vi "4Pi Interference Locator NEW.vi"(7 "Calling VI Ref":refnum<vi>) -> ()   [LabVIEW 2016]
uses:
  <vilib>/vision/Image Controls.llb/IMAQ Image.ctl
  Hardware Configuration/Hardware Configuration Controls/Device Type.ctl
  Hardware Configuration/Hardware Configuration Controls/Device Function.ctl
  Device Library/Stages/Stages Controls/Stage Actions.ctl
  <vilib>/Utility/miscctls.llb/LVPointTypeDef.ctl
  4Pi Interference Locator Type Defs/4Pi IL Notifier Type.ctl
  4Pi Interference Locator Type Defs/4Pi IL Actions.ctl
  Device Manager/Common Device Queue/Common Device Controls/Common Device Actions.ctl
  Device Library/Cameras/Hamamatsu/Orca Flash/Orca Flash Controls/Orca Flash Actions.ctl
  Display Module/Display Module Custom Controls/ROI Descriptor.ctl
  Device Library/Stages/Stages Controls/Stage Status.ctl
  <vilib>/vision/NI_Vision_Development_Module.lvlib
panel:
  in  "Move to Cursor":bool
  in  "Halt Stage":bool
  in  "Scan Range (µm)":dbl
  out "Interference Scan":cluster{sgl[], sgl[]}(graph)
  in  "Clear Plot":bool=TRUE
  in  "Stage Settings":bool
  in  "Scan Cavity":bool
  in  "Velocity":dbl=0.001
  in  "Quit":bool
  in  "Interference Image":i32(ring) items=["Quad 01", "Quad 02", "Quad 03", "Quad 04"]
  in  "Cavity Position (µm)":dbl
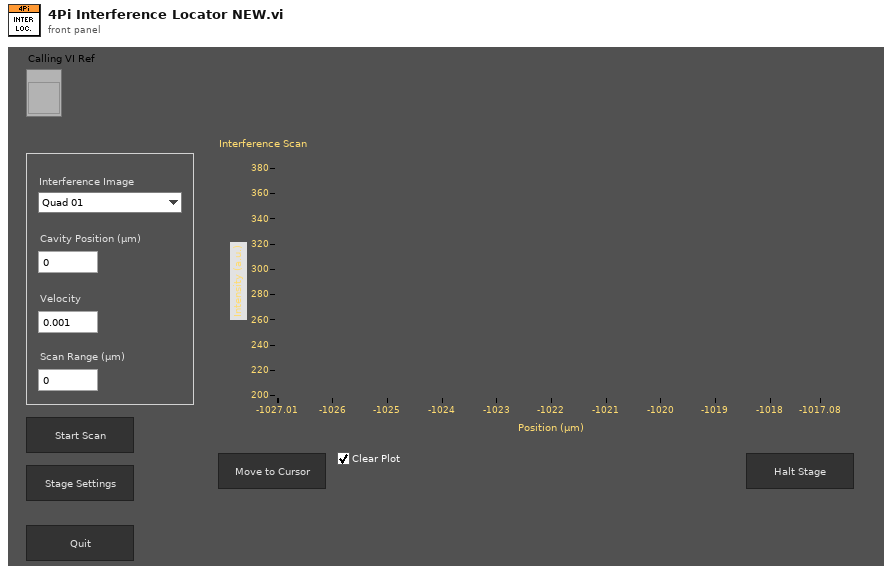
[diagram p1: front panel]
types:
  T1 = typedef "4Pi IL Actions.ctl" = enum16{"Idle", "Start Scan", "Move Stage", "Get Data", "Wait For Update", "Abort", "End Scan", "Quit"}
  T2 = typedef "4Pi IL Notifier Type.ctl" = cluster{"Actions":T1, "Image Ref":T3, "Scan Image Mask":T3}
  T3 = typedef "IMAQ Image.ctl" = refnum<image>
  T4 = enum16{"Always On", "Always Off", "Off While Running"}
  T5 = typedef "LVPointTypeDef.ctl" = cluster{"Horizontal":i16, "Vertical":i16}
  T6 = typedef "Stage Actions.ctl" = enum16{"Get Position", "MVR", "MOVE", "HALT", "ONTARGET", "ERROR", "REFERENCE", "INIT", "VELOCITY", "STATUS", "EXIT", "HOME", "ZEROPOS", "NANOPOS", "ANALOG", "QUIT"}
  T7 = typedef "Image Type" = u32
  T8 = typedef "Device Function.ctl" = enum16{"Primary", "Secondary", "Overview", "Wide Field Drift Correction", "642 nm Excitation", "560 nm Excitation", "546 nm Excitation", "488 nm Excitation", "405 nm Excitation", "Objective Drift Correction", "Objective XY", "Objective Z", "Sample XY", "Sample Coarse Z", "Sample Z", "4Pi Lower", "4Pi Upper", "Adj Cavity", "Line Scanning"}
  T9 = typedef "Device Type.ctl" = enum16{"AOTF", "Camera", "Deformable Mirror", "Laser", "Shutter", "Stage", "Waveform"}
  T10 = typedef "ROI Descriptor.ctl" = cluster{"Global Rectangle":i32[], "Contours":cluster{"Contour Type":u32, "ROI Type":u32, "Points":i32[]}[]}
  T11 = typedef "Orca Flash Actions.ctl" = enum16{"IDLE", "PREVIEW", "RECORD", "Record Settings", "SETPARAM", "GETPARAM", "SETROI", "GETROI", "PROGRESSIVE MODE", "AREA MODE", "STATUS", "QUIT"}
  T12 = typedef "Stage Status.ctl" = enum16{"Error", "Abort", "Busy", "On Target"}
  T13 = typedef "Common Device Actions.ctl" = enum16{"Open Front Panel", "Close Front Panel", "Quit", "Quit All"}
  T14 = cluster{"Contour Type":u32, "ROI Type":u32, "Points":i32[]}[]
  T15 = cluster{"Contour Type":u32, "ROI Type":u32, "Points":i32[]}
  T16 = cluster{"Mean Value":sgl, "Standard Variation":sgl, "Minimal Value":sgl, "Maximal Value":sgl, "Area (calibrated)":sgl, "Area (pixels)":u32, "%":sgl, "Calibration Valid":bool}
  T17 = typedef "LVRectTypeDef.ctl" = cluster{"Left":i16, "Top":i16, "Right":i16, "Bottom":i16}
  T18 = typedef "LVBoundsTypeDef.ctl" = cluster{"Width":u32, "Height":u32}
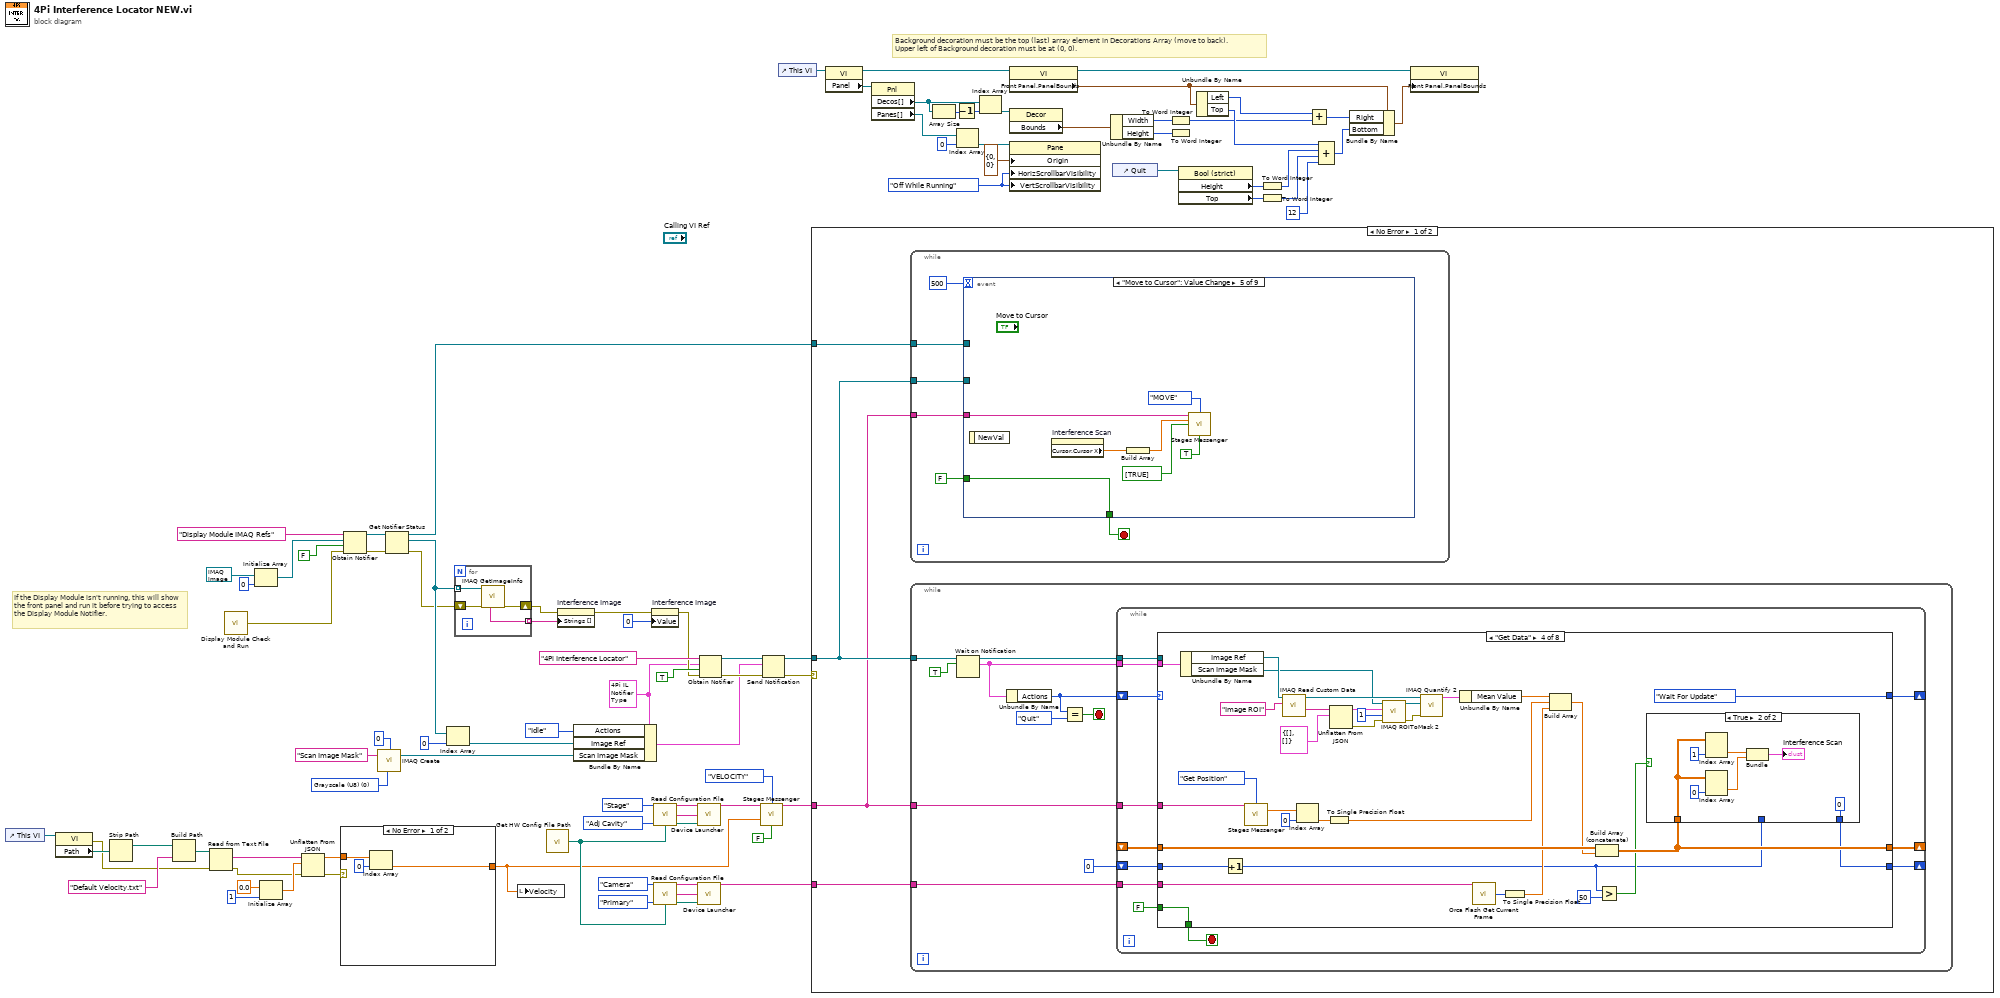
[diagram p0: block diagram]
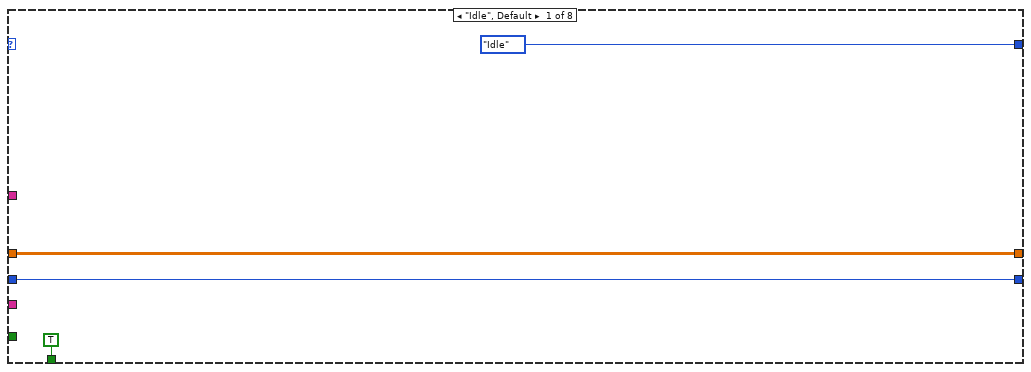
[diagram p2: hidden frame]
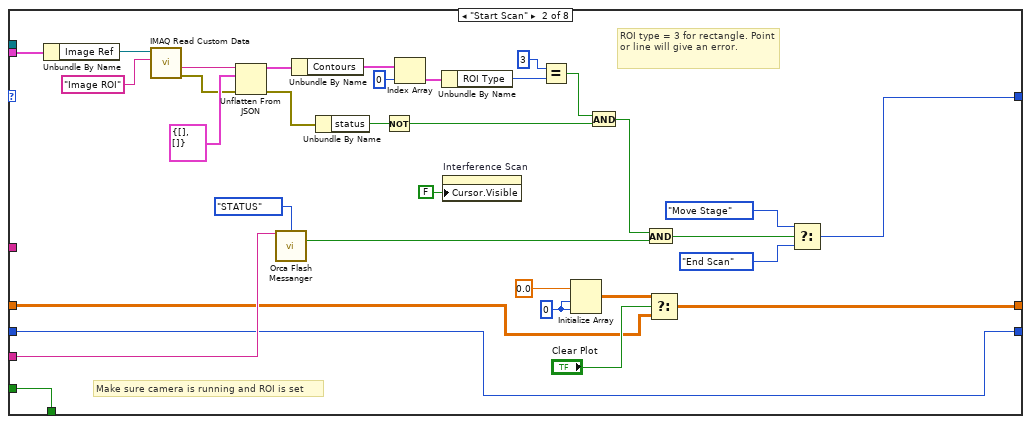
[diagram p3: hidden frame]
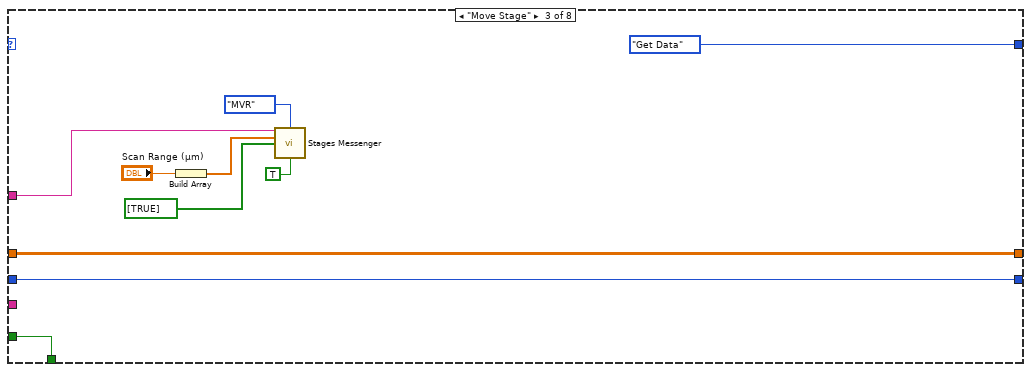
[diagram p4: hidden frame]
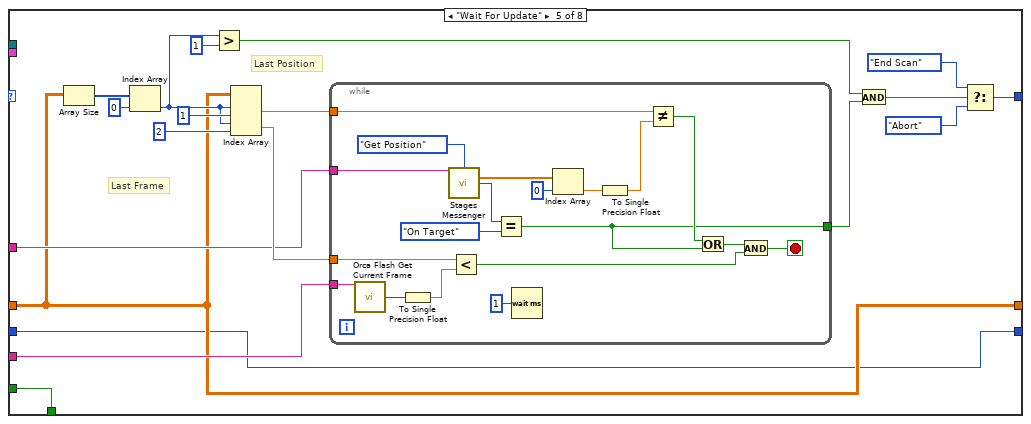
[diagram p6: hidden frame]
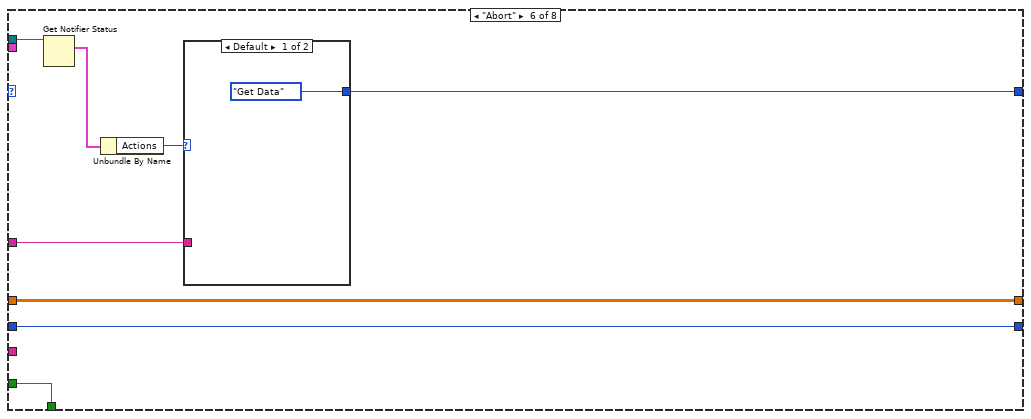
[diagram p7: hidden frame]
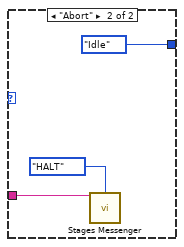
[diagram p8: hidden frame]
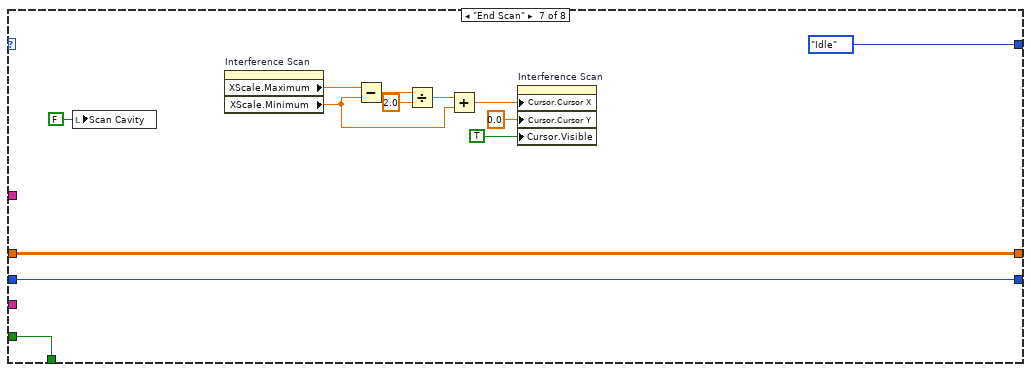
[diagram p9: hidden frame]
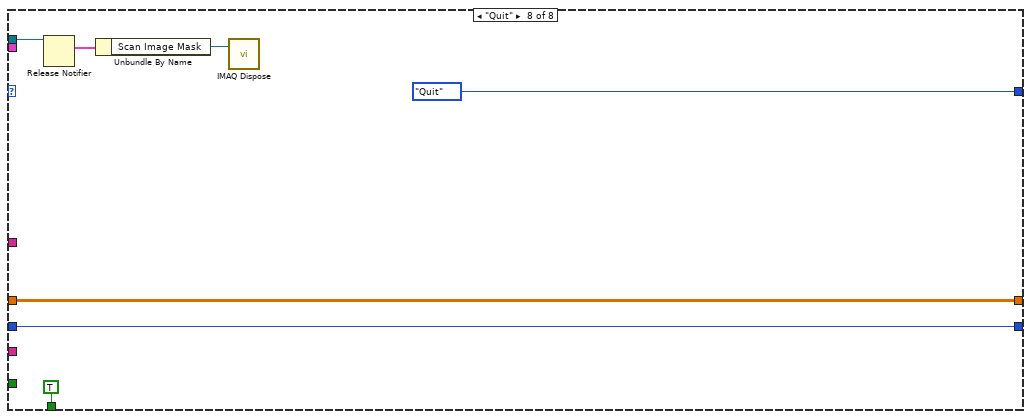
[diagram p10: hidden frame]
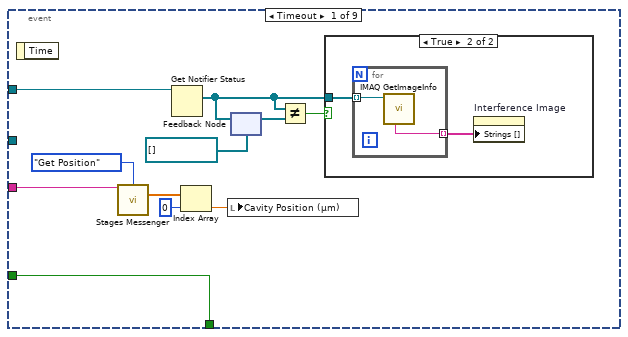
[diagram p11: hidden frame]
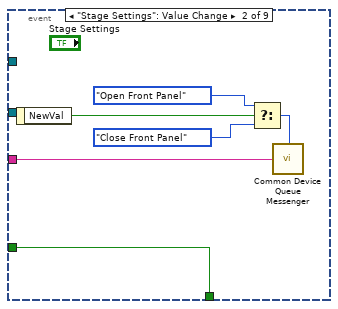
[diagram p13: hidden frame]
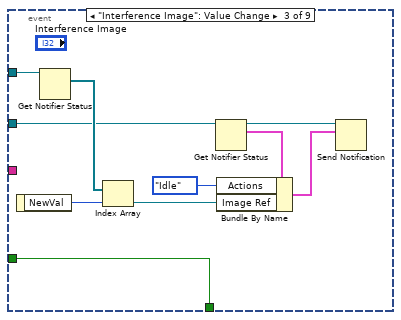
[diagram p14: hidden frame]
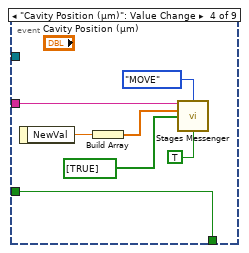
[diagram p15: hidden frame]
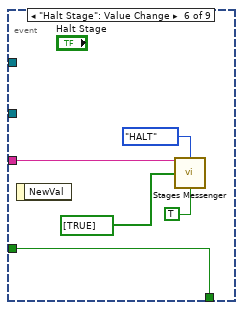
[diagram p16: hidden frame]
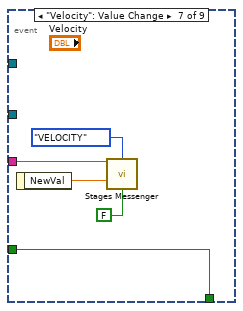
[diagram p17: hidden frame]
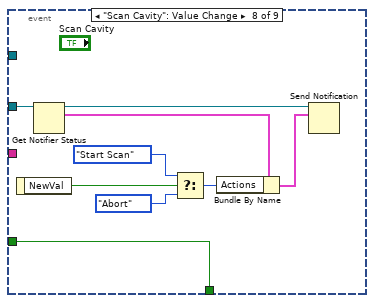
[diagram p18: hidden frame]
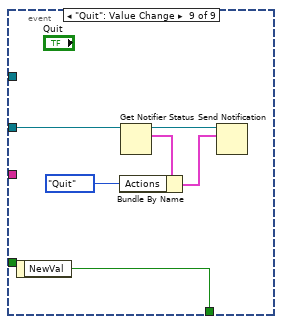
[diagram p19: hidden frame]
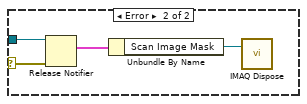
[diagram p20: hidden frame]
diagram:
  w9 = T2 {"Actions"=enum."Idle", "Image Ref"=refnum, "Scan Image Mask"=refnum} ("4Pi IL Notifier Type")
  w49 = T4."Off While Running" ("Vertical Scrollbar Visibility")
  w71 = T7 0 items=["Grayscale (U8)", "Grayscale (I16)", "Grayscale (SGL)", "Complex (CSG)", "RGB (U32)", "HSL (U32)", "RGB (U64)", "Grayscale (U16)"] ("Image Type")
  # "If the Display Module isn't running, this will show the front panel and run it before trying to access the Display Module Notifier."
  # "Background decoration must be the top (last) array element in Decorations Array (move to back).\nUpper left of Background decoration must be at (0, 0)."
  n1 = control-ref of="This VI"() -> (w37:refnum<vi>)
  n2 = property class="VI"(reference=w37) -> (error out=w28:errorcluster, "Path"=w36:path)  [unwired: 1 in, 1 out]
  n3 = Strip Path(path=w36) -> (stripped path=w29:path)  [unwired: 1 out]
  n4 = Build Path(base path=w29, name or relative path="Default Velocity.txt") -> (appended path=w31:path)
  n5 = Read from Text File(file (use dialog)=w31, error in=w28) -> (text=w30:string, error out=w27:errorcluster)  [unwired: 2 in, 2 out]
  n6 = call "Display Module Check and Run.vi"() -> ("Error"=w23:errorcluster)  [unwired: 15 in]
  n7 = Initialize Array(T3 refnum ("New Image"), 0 ("dimension size")) -> (w86:T3[])
  n8 = Initialize Array(0.0 ("element"), 1 ("dimension size")) -> (w32:dbl[])
  n9 = Unflatten From JSON(JSON string=w30, type and defaults=w32, error in (no error)=w27) -> (value=w25:dbl[], error out=w26:errorcluster)  [unwired: 4 in]
  n10 = case shown="No Error" w26 {
    tunnel: w25 -> [w92 _]
    tunnel: [w91 1.0 ("element")] -> w24
    frame No Error {
      n11 = Index Array(array=w92, index=0) -> (element=w91:dbl)
    }
    frame Error {
      n12 = One Button Dialog(message="Default cavity stage velocity not found in 4Pi Interference Locator. Please set this value") -> ()  [unwired: 1 in, 1 out]
    }
  }
  n13 = Obtain Notifier(name (unnamed)="Display Module IMAQ Refs", notification data type=w86, create if not found? (T)=FALSE, error in (no error)=w23) -> (notifier out=w85:refnum<notifier>, error out=w22:errorcluster)  [unwired: 1 out]
  n14 = call "IMAQ Create"("Border Size"=0, "Image Name"="Scan Image Mask", "Image Type"=w71) -> ("New Image"=w1:T3)  [unwired: 2 in, 1 out]
  n15 = Get Notifier Status(notifier=w85, error in (no error)=w22) -> (notifier out=w2:refnum<notifier>, current notification=w20:T3[], error out=w19:errorcluster)  [unwired: 2 out]
  n16 = Index Array(array=w20, index=0) -> (element=w7:T3)
  n17 = for {
    tunnel: w20 -> [w99] mode=indexing
    shift-right: [w97] -> w14
    shift-left: w19 -> [w98]
    tunnel: [w96] -> w18 mode=indexing
    n18 = call "IMAQ GetImageInfo"("error in (no error)"=w98, "Image"=w99) -> ("error out"=w97:errorcluster, "Image Name"=w96:string)  [unwired: 2 in, 6 out]
  }
  n19 = local write "Velocity"(w24) -> ()
  n20 = call "Get HW Config File Path.vi"() -> ("File Path"=w73:path)  [unwired: 14 in, 1 out]
  n21 = property on="Interference Image" class="Ring (strict)"(error in=w14, "Strings []"=w18) -> (error out=w21:errorcluster)  [unwired: 1 in, 1 out]
  n22 = Bundle By Name(cluster=w9, "Actions"=4Pi_IL_Actions."Idle", "Image Ref"=w7, "Scan Image Mask"=w1) -> (w6:T2)
  n23 = property on="Interference Image" class="Ring (strict)"(error in=w21, "Value"=0) -> (error out=w13:errorcluster)  [unwired: 1 in, 1 out]
  n24 = call "Read Configuration File.vi"("Device Type"=Device_Type."Stage", "Device Function"=Device_Function."Adj Cavity", "Config File Path"=w73) -> ("Unique Notifier Name"=w83:string, "Device Ports/IDs/Channels"=w81:string[], "Device Engine Path"=w82:path)  [unwired: 9 in, 1 out]
  n25 = call "Read Configuration File.vi"("Device Type"=Device_Type."Camera", "Device Function"=Device_Function."Primary", "Config File Path"=w73) -> ("Unique Notifier Name"=w74:string, "Device Ports/IDs/Channels"=w76:string[], "Device Engine Path"=w75:path)  [unwired: 9 in, 1 out]
  n26 = call "Device Launcher.vi"("Notifier Name"=w83, "Device Ports/IDs/Channels"=w81, "Device Engine Path"=w82) -> ("Notifier Name"=w67:string)  [unwired: 11 in, 1 out]
  n27 = call "Device Launcher.vi"("Notifier Name"=w74, "Device Ports/IDs/Channels"=w76, "Device Engine Path"=w75) -> ("Notifier Name"=w3:string)  [unwired: 11 in, 1 out]
  n28 = Obtain Notifier(name (unnamed)="4Pi Interference Locator", notification data type=w9, create if not found? (T)=TRUE, error in (no error)=w13) -> (notifier out=w12:refnum<notifier>, error out=w11:errorcluster)  [unwired: 1 out]
  n29 = call "Stages Messenger.vi"("Stage Notifier Name"=w67, "Actions"=Stage_Actions."VELOCITY", "Velocity"=w24, "Exit While Busy?"=FALSE) -> ("Stage Notifier Name (Dup)"=w4:string)  [unwired: 8 in, 3 out]
  n30 = Send Notification(notification=w6, notifier=w12, error in (no error)=w11) -> (notifier out=w5:refnum<notifier>, error out=w10:errorcluster)
  n31 = control-ref of="This VI"() -> (w41:refnum<vi>)
  n32 = case shown="No Error" w10 {
    selector: w10 -> [_ w361]
    tunnel: w5 -> [w103 w362]
    tunnel: w4 -> [w101 _]
    tunnel: w3 -> [w102 _]
    tunnel: w2 -> [w100 _]
    frame No Error {
      n33 = while {
        tunnel: w103 -> [w286]
        tunnel: w101 -> [w285]
        tunnel: w100 -> [w284]
        stop <- w288 stop-if-true
        n34 = event shown="[4] \"Move to Cursor\": Value Change" {
          selector: _ -> [_ _ _ _ _ _ _ _ _]
          dyn-events: _ -> [_ _ _ _ _ _ _ _ _]
          timeout: 500 -> [_ _ _ _ _ _ _ _ _]
          tunnel: w284 -> [w300 _ w319 _ _ _ _ _ _]
          tunnel: [w296 w310 w320 w327 w334 w339 w344 w348 w359] -> w288
          tunnel: FALSE -> [w296 w310 w320 w327 w334 w339 w344 w348 _]
          tunnel: w285 -> [w295 w306 _ w324 w332 w337 w341 _ _]
          tunnel: w286 -> [_ _ w316 _ _ _ _ w352 w358]
          event Timeout {
            n35 = event-data() -> ()  [unwired: 1 in, 1 out]
            n36 = call "Stages Messenger.vi"("Stage Notifier Name"=w295, "Actions"=Stage_Actions."Get Position") -> ("Positions"=w293:dbl[])  [unwired: 10 in, 3 out]
            n37 = Get Notifier Status(notifier=w300) -> (current notification=w297:T3[])  [unwired: 1 in, 4 out]
            n38 = Index Array(array=w293, index=0) -> (element=w291:dbl)
            n39 = local write "Cavity Position (µm)"(w291) -> ()
            n40 = feedback-in #1(w297) -> ()
            n41 = feedback #1(T3[] []) -> (w299:T3[])
            n42 = Not Equal?(x=w297, y=w299) -> (x != y?=w298:bool)
            n43 = case shown="True" w298 {
              tunnel: w297 -> [_ w302]
              frame False {
              }
              frame True {
                n44 = for {
                  tunnel: w302 -> [w304] mode=indexing
                  tunnel: [w303] -> w301 mode=indexing
                  n45 = call "IMAQ GetImageInfo"("Image"=w304) -> ("Image Name"=w303:string)  [unwired: 3 in, 7 out]
                }
                n46 = property on="Interference Image" class="Ring (strict)"("Strings []"=w301) -> ()  [unwired: 2 in, 2 out]
              }
            }
          }
          event "Stage Settings": Value Change {
            n47 = event-data() -> ("NewVal"=w305:bool)  [unwired: 1 in]
            n48 = Select(t=Common_Device_Actions."Open Front Panel" ("Common Actions"), s=w305, f=Common_Device_Actions."Close Front Panel" ("Common Actions")) -> (s? t:f=w309:T13)
            n49 = call "Common Device Queue Messenger.vi"("Common Action"=w309, "Notifier Name"=w306) -> ()  [unwired: 13 in, 1 out]
          }
          event "Interference Image": Value Change {
            n50 = event-data() -> ("NewVal"=w317:i32)  [unwired: 1 in]
            n51 = Get Notifier Status(notifier=w319) -> (current notification=w318:T3[])  [unwired: 1 in, 4 out]
            n52 = Index Array(array=w318, index=w317) -> (element=w313:T3)
            n53 = Get Notifier Status(notifier=w316) -> (notifier out=w312:refnum<notifier>, current notification=w315:T2)  [unwired: 1 in, 3 out]
            n54 = Bundle By Name(cluster=w315, "Actions"=4Pi_IL_Actions."Idle", "Image Ref"=w313) -> (w311:T2)
            n55 = Send Notification(notification=w311, notifier=w312) -> ()  [unwired: 1 in, 2 out]
          }
          event "Cavity Position (µm)": Value Change {
            n56 = event-data() -> ("NewVal"=w326:dbl)  [unwired: 1 in]
            n57 = Build Array(w326) -> (w323:dbl[])
            n58 = call "Stages Messenger.vi"("Stage Notifier Name"=w324, "Actions"=Stage_Actions."MOVE", "Setpoint"=w323, "Axis"=bool[] [TRUE], "Exit While Busy?"=TRUE) -> ()  [unwired: 7 in, 4 out]
          }
          event "Move to Cursor": Value Change {
            n59 = event-data() -> ()  [unwired: 1 in, 1 out]
            n60 = property on="Interference Scan" class="XYGraph (strict)"() -> ("Cursor.Cursor X"=w328:dbl)  [unwired: 2 in, 2 out]
            n61 = Build Array(w328) -> (w331:dbl[])
            n62 = call "Stages Messenger.vi"("Stage Notifier Name"=w332, "Actions"=Stage_Actions."MOVE", "Setpoint"=w331, "Axis"=bool[] [TRUE], "Exit While Busy?"=TRUE) -> ()  [unwired: 7 in, 4 out]
          }
          event "Halt Stage": Value Change {
            n63 = event-data() -> ()  [unwired: 1 in, 1 out]
            n64 = call "Stages Messenger.vi"("Stage Notifier Name"=w337, "Actions"=Stage_Actions."HALT", "Axis"=bool[] [TRUE], "Exit While Busy?"=TRUE) -> ()  [unwired: 8 in, 4 out]
          }
          event "Velocity": Value Change {
            n65 = event-data() -> ("NewVal"=w340:dbl)  [unwired: 1 in]
            n66 = call "Stages Messenger.vi"("Stage Notifier Name"=w341, "Actions"=Stage_Actions."VELOCITY", "Velocity"=w340, "Exit While Busy?"=FALSE) -> ()  [unwired: 8 in, 4 out]
          }
          event "Scan Cavity": Value Change {
            n67 = event-data() -> ("NewVal"=w353:bool)  [unwired: 1 in]
            n68 = Get Notifier Status(notifier=w352) -> (notifier out=w345:refnum<notifier>, current notification=w351:T2)  [unwired: 1 in, 3 out]
            n69 = Select(t=4Pi_IL_Actions."Start Scan" ("Actions"), s=w353, f=4Pi_IL_Actions."Abort" ("Actions")) -> (s? t:f=w347:T1)
            n70 = Bundle By Name(cluster=w351, "Actions"=w347) -> (w346:T2)
            n71 = Send Notification(notification=w346, notifier=w345) -> ()  [unwired: 1 in, 2 out]
          }
          event "Quit": Value Change {
            n72 = event-data() -> ("NewVal"=w359:bool)  [unwired: 1 in]
            n73 = Get Notifier Status(notifier=w358) -> (notifier out=w357:refnum<notifier>, current notification=w356:T2)  [unwired: 1 in, 3 out]
            n74 = Bundle By Name(cluster=w356, "Actions"=4Pi_IL_Actions."Quit") -> (w354:T2)
            n75 = Send Notification(notification=w354, notifier=w357) -> ()  [unwired: 1 in, 2 out]
          }
        }
      }
      n76 = while {
        tunnel: w103 -> [w113]
        tunnel: w101 -> [w105]
        tunnel: w102 -> [w106]
        stop <- w109 stop-if-true
        n77 = Wait on Notification(notifier=w113, ignore previous (F)=TRUE) -> (notifier out=w107:refnum<notifier>, notification=w108:T2)  [unwired: 2 in, 2 out]
        n78 = Unbundle By Name(w108) -> ("Actions"=w110:T1)
        n79 = Equal?(x=w110, y=4Pi_IL_Actions."Quit") -> (x = y?=w109:bool)
        n80 = while {
          tunnel: w108 -> [w124]
          tunnel: w107 -> [w123]
          tunnel: w106 -> [w122]
          shift-right: [w121] -> _
          shift-left: w110 -> [w125]
          shift-right: [w118] -> _
          shift-left: _ -> [w117]
          tunnel: w105 -> [w116]
          shift-right: [w114] -> _
          shift-left: u8 0 -> [w115]
          stop <- w119 stop-if-true
          n81 = case shown="\"Get Data\"" w125 {
            tunnel: w124 -> [_ w160 _ w204 _ _ _ _]
            tunnel: w123 -> [_ _ _ _ _ w257 _ w283]
            tunnel: w122 -> [_ w159 _ w180 w225 _ _ _]
            tunnel: [4Pi_IL_Actions."Idle" ("f") w156 4Pi_IL_Actions."Get Data" ("f") 4Pi_IL_Actions."Wait For Update" ("f") w222 w253 4Pi_IL_Actions."Idle" ("f") 4Pi_IL_Actions."Quit" ("f")] -> w121
            tunnel: FALSE -> [_ w154 w172 w205 w232 w259 w275 _]
            tunnel: [TRUE w154 w172 w205 w232 w259 w275 TRUE] -> w119
            tunnel: [w127 w149 w171 w183 w215 w258 w276 w280] -> w118
            tunnel: w117 -> [w127 w148 w171 w185 w215 w258 w276 w280]
            tunnel: w116 -> [_ _ w165 w188 w224 w254 _ _]
            tunnel: w115 -> [w126 w130 w163 w177 w214 w252 w264 w277]
            tunnel: [w126 w130 w163 w173 w214 w252 w264 w277] -> w114
            frame "Idle", Default {
            }
            frame "Start Scan" {
              w151 = 0 ("dimension size")
              # "ROI type = 3 for rectangle. Point or line will give an error."
              # "Make sure camera is running and ROI is set"
              n82 = Unbundle By Name(w160) -> ("Image Ref"=w144:T3)
              n83 = call "IMAQ Read Custom Data"("Key"="Image ROI", "Image"=w144) -> ("error out"=w143:errorcluster, "Custom Data Out"=w146:string)  [unwired: 7 in, 1 out]
              n84 = Unflatten From JSON(JSON string=w146, type and defaults=T10 {"Global Rectangle"=[], "Contours"=[]} ("Image ROI Descriptor"), error in (no error)=w143) -> (value=w137:T10, error out=w136:errorcluster)  [unwired: 4 in]
              n85 = call "Orca Flash Messanger.vi"("Notifier Name"=w159, "Camera Actions"=Orca_Flash_Actions."STATUS") -> ("Running?"=w161:bool)  [unwired: 9 in, 4 out]
              n86 = Unbundle By Name(w137) -> ("Contours"=w138:T14)
              n87 = Unbundle By Name(w136) -> ("status"=w135:bool)
              n88 = Not(x=w135) -> (.not. x?=w133:bool)
              n89 = Index Array(array=w138, index=0) -> (element=w140:T15)
              n90 = Unbundle By Name(w140) -> ("ROI Type"=w141:u32)
              n91 = property on="Interference Scan" class="XYGraph (strict)"("Cursor.Visible"=FALSE) -> ()  [unwired: 2 in, 2 out]
              n92 = Equal?(x=u32 3, y=w141) -> (x = y?=w134:bool)
              n93 = Initialize Array(sgl 0.0, w151, w151) -> (w150:sgl[][])
              n94 = And(x=w134, y=w133) -> (x .and. y?=w132:bool)
              n95 = And(x=w132, y=w161) -> (x .and. y?=w158:bool)
              n96 = Select(t=w150, s="Clear Plot", f=w148) -> (s? t:f=w149:sgl[][])
              n97 = Select(t=4Pi_IL_Actions."Move Stage" ("y"), s=w158, f=4Pi_IL_Actions."End Scan") -> (s? t:f=w156:T1)
            }
            frame "Move Stage" {
              n98 = Build Array("Scan Range (µm)") -> (w168:dbl[])
              n99 = call "Stages Messenger.vi"("Stage Notifier Name"=w165, "Actions"=Stage_Actions."MVR", "Setpoint"=w168, "Axis"=bool[] [TRUE], "Exit While Busy?"=TRUE) -> ()  [unwired: 7 in, 4 out]
            }
            frame "Get Data" {
              n100 = Unbundle By Name(w204) -> ("Image Ref"=w193:T3, "Scan Image Mask"=w192:T3)
              n101 = Increment(x=w177) -> (x+1=w174:u8)
              n102 = call "Stages Messenger.vi"("Stage Notifier Name"=w188, "Actions"=Stage_Actions."Get Position") -> ("Positions"=w191:dbl[])  [unwired: 10 in, 3 out]
              n103 = call "IMAQ Read Custom Data"("Key"="Image ROI", "Image"=w193) -> ("Custom Data Out"=w202:string, "Image (duplicate)"=w194:T3)  [unwired: 7 in, 1 out]
              n104 = Index Array(array=w191, index=0) -> (element=w187:dbl)
              n105 = To Single Precision Float(number=w187) -> (single precision float=w186:sgl)
              n106 = Unflatten From JSON(JSON string=w202, type and defaults=T10 {"Global Rectangle"=[], "Contours"=[]} ("Image ROI Descriptor")) -> (value=w200:T10, error out=w196:errorcluster)  [unwired: 5 in]
              n107 = call "IMAQ ROIToMask 2"("error in (no error)"=w196, "Filling Value (255)"=1, "ROI Descriptor"=w200, "Image"=w192) -> ("error out"=w197:errorcluster, "Image Out"=w198:T3)  [unwired: 5 in, 1 out]
              n108 = call "IMAQ Quantify 2"("error in (no error)"=w197, "Image Mask"=w198, "Image"=w194) -> ("Global Report"=w195:T16)  [unwired: 6 in, 2 out]
              n109 = Unbundle By Name(w195) -> ("Mean Value"=w181:sgl)
              n110 = call "Orca Flash Get Current Frame.vi"("Camera Notifier Name"=w180) -> ("Current Frame"=w179:u32)  [unwired: 13 in, 1 out]
              n111 = To Single Precision Float(number=w179) -> (single precision float=w178:sgl)
              n112 = Build Array(w181, w186, w178) -> (w184:sgl[])
              n113 = Build Array (concatenate)(w185, w184) -> (w183:sgl[][])
              n114 = Greater?(x=w174, y=u8 50) -> (0:w175:bool)
              n115 = case shown="True" w175 {
                tunnel: w183 -> [_ w209]
                tunnel: w174 -> [w206 _]
                tunnel: [w206 u8 0] -> w173
                frame False {
                }
                frame True {
                  n116 = Index Array(array=w209, index (col)=1 ("disabled index (col)")) -> (element=w211:sgl[])  [unwired: 1 in]
                  n117 = Index Array(array=w209, index (col)=0 ("disabled index (col)")) -> (element=w210:sgl[])  [unwired: 1 in]
                  n118 = Bundle(w211, w210) -> (→"Interference Scan":cluster{sgl[], sgl[]})  [unwired: 1 in]
                }
              }
            }
            frame "Wait For Update" {
              # "Last Frame"
              # "Last Position"
              n119 = Array Size(array=w215) -> (size(s)=w231:i32[])
              n120 = Index Array(array=w231, index=0) -> (element=w220:i32)
              n121 = Greater?(x=w220, y=1) -> (0:w217:bool)
              n122 = Index Array(array=w215, index (row) #1=w220, index (col) #1=1 ("disabled index (col)"), index (row) #2=w220, index (col) #2=2 ("disabled index (col)")) -> (element #1=w227:sgl, element #2=w226:sgl)
              n123 = while {
                tunnel: w226 -> [w249]
                tunnel: w225 -> [w248]
                tunnel: w224 -> [w244]
                tunnel: w227 -> [w243]
                tunnel: [w233] -> w218
                stop <- w235 stop-if-true
                n124 = call "Orca Flash Get Current Frame.vi"("Camera Notifier Name"=w248) -> ("Current Frame"=w251:u32)  [unwired: 13 in, 1 out]
                n125 = To Single Precision Float(number=w251) -> (single precision float=w250:sgl)
                n126 = call "Stages Messenger.vi"("Stage Notifier Name"=w244, "Actions"=Stage_Actions."Get Position") -> ("Positions"=w242:dbl[], "Status"=w246:T12)  [unwired: 10 in, 2 out]
                n127 = Less?(x=w249, y=w250) -> (x < y?=w236:bool)
                n128 = Equal?(x=w246, y=Stage_Status."On Target") -> (x = y?=w233:bool)
                n129 = Wait (ms)(milliseconds to wait=u32 1) -> ()  [unwired: 1 out]
                n130 = Index Array(array=w242, index=0) -> (element=w240:dbl)
                n131 = To Single Precision Float(number=w240) -> (single precision float=w239:sgl)
                n132 = Not Equal?(x=w243, y=w239) -> (x != y?=w238:bool)
                n133 = Or(x=w238, y=w233) -> (x .or. y?=w237:bool)
                n134 = And(x=w237, y=w236) -> (x .and. y?=w235:bool)
              }
              n135 = And(x=w217, y=w218) -> (x .and. y?=w216:bool)
              n136 = Select(t=4Pi_IL_Actions."End Scan" ("y"), s=w216, f=4Pi_IL_Actions."Abort" ("y")) -> (s? t:f=w222:T1)
            }
            frame "Abort" {
              n137 = Get Notifier Status(notifier=w257) -> (current notification=w256:T2)  [unwired: 1 in, 4 out]
              n138 = Unbundle By Name(w256) -> ("Actions"=w255:T1)
              n139 = case shown="Default" w255 {
                tunnel: w254 -> [_ w263]
                tunnel: [4Pi_IL_Actions."Get Data" ("f") 4Pi_IL_Actions."Idle" ("f")] -> w253
                frame Default {
                }
                frame "Abort" {
                  n140 = call "Stages Messenger.vi"("Stage Notifier Name"=w263, "Actions"=Stage_Actions."HALT") -> ()  [unwired: 10 in, 4 out]
                }
              }
            }
            frame "End Scan" {
              n141 = local write "Scan Cavity"(FALSE ("Scan Cavity")) -> ()
              n142 = property on="Interference Scan" class="XYGraph (strict)"() -> ("XScale.Maximum"=w272:dbl, "XScale.Minimum"=w265:dbl)  [unwired: 2 in, 2 out]
              n143 = Subtract(x=w272, y=w265) -> (x-y=w269:dbl)
              n144 = Divide(x=w269, y=2.0) -> (x/y=w267:dbl)
              n145 = Add(x=w267, y=w265) -> (x+y=w266:dbl)
              n146 = property on="Interference Scan" class="XYGraph (strict)"("Cursor.Cursor X"=w266, "Cursor.Cursor Y"=0.0 ("Cursor.Cursor Position:Cursor Y"), "Cursor.Visible"=TRUE) -> ()  [unwired: 2 in, 2 out]
            }
            frame "Quit" {
              n147 = Release Notifier(notifier=w283) -> (last notification=w278:T2)  [unwired: 2 in, 2 out]
              n148 = Unbundle By Name(w278) -> ("Scan Image Mask"=w279:T3)
              n149 = call "IMAQ Dispose"("Image"=w279) -> ()  [unwired: 5 in, 1 out]
            }
          }
        }
      }
    }
    frame Error {
      n150 = Release Notifier(notifier=w362, error in (no error)=w361) -> (last notification=w360:T2)  [unwired: 1 in, 2 out]
      n151 = Unbundle By Name(w360) -> ("Scan Image Mask"=w363:T3)
      n152 = call "IMAQ Dispose"("Image"=w363) -> ()  [unwired: 5 in, 1 out]
    }
  }
  n153 = property class="VI"(reference=w41) -> (reference out=w50:refnum<vi>, "Panel"=w42:refnum<vi>)  [unwired: 1 in, 1 out]
  n154 = property class="Pnl"(reference=w42) -> ("Decos[]"=w40:refnum<vi>[], "Panes[]"=w46:refnum<vi>[])  [unwired: 1 in, 2 out]
  n155 = Array Size(array=w40) -> (size(s)=w38:i32)
  n156 = Decrement(x=w38) -> (x-1=w39:i32)
  n157 = Index Array(array=w46, index=0) -> (element=w45:refnum<vi>)
  n158 = Index Array(array=w40, index=w39) -> (element=w48:refnum<vi>)
  n159 = property class="VI"(reference=w50) -> (reference out=w52:refnum<vi>, "Front Panel.PanelBounds"=w53:T17)  [unwired: 1 in, 1 out]
  n160 = property class="Decor"(reference=w48) -> ("Bounds"=w51:T18)  [unwired: 1 in, 2 out]
  n161 = property class="Pane"(reference=w45, "Origin"=T5 {"Horizontal"=0, "Vertical"=0}, "HorizScrollbarVisibility"=w49, "VertScrollbarVisibility"=w49) -> ()  [unwired: 1 in, 2 out]
  n162 = Unbundle By Name(w51) -> ("Width"=w56:u32, "Height"=w59:u32)
  n163 = control-ref of="Quit"() -> (w43:refnum<vi>)
  n164 = To Word Integer(number=w56) -> (16bit integer=w58:i16)
  n165 = To Word Integer(number=w59) -> ()  [unwired: 1 out]
  n166 = property class="Bool (strict)"(reference=w43) -> ("Height"=w61:u32, "Top"=w62:i32)  [unwired: 1 in, 2 out]
  n167 = Unbundle By Name(w53) -> ("Left"=w55:i16, "Top"=w66:i16)
  n168 = To Word Integer(number=w61) -> (16bit integer=w64:i16)
  n169 = To Word Integer(number=w62) -> (16bit integer=w65:i16)
  n170 = Add(x=w55, y=w58) -> (x+y=w57:i16)
  n171 = Compound Arithmetic op=ADD(w66, w64, w65, i16 12 ("y")) -> (w60:i16)
  n172 = Bundle By Name(cluster=w53, "Right"=w57, "Bottom"=w60) -> (w54:T17)
  n173 = property class="VI"(reference=w52, "Front Panel.PanelBounds"=w54) -> ()  [unwired: 1 in, 2 out]
